vi "Zero-Pole (DBL).vi"(2 "initialize":bool, 3 "dt":dbl=1e-09 min=1e-09 format="%.6f", 4 "gain-zeros-poles":T1 {"Poles" format="%.2f"; "Zeros" format="%.2f"; "gain" format="%.2f"}, 5 "input point":dbl format="%.2f") -> (1 "output point":dbl format="%.2f")   [LabVIEW 2017, in "NI_AdvCtrl_continuous linear.lvlib"]
doc: "LabVIEW no longer supports this VI. You can obtain similar functionality by installing the LabVIEW Simulation Module.\n\nCalculates the new output point, where the transfer function and the input point are given. The transfer function is described in gain-zeros-poles notation."
uses:
  <vilib>/addons/control/advanced/NI_AdvCtrl_continuous linear.lvlib
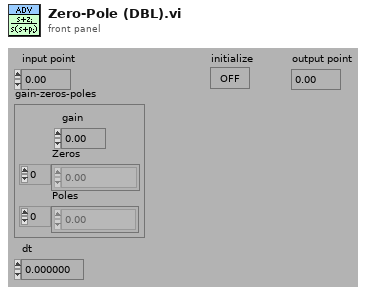
[diagram p1: front panel]
types:
  T1 = cluster{"gain":dbl, "Zeros":cdb[], "Poles":cdb[]}
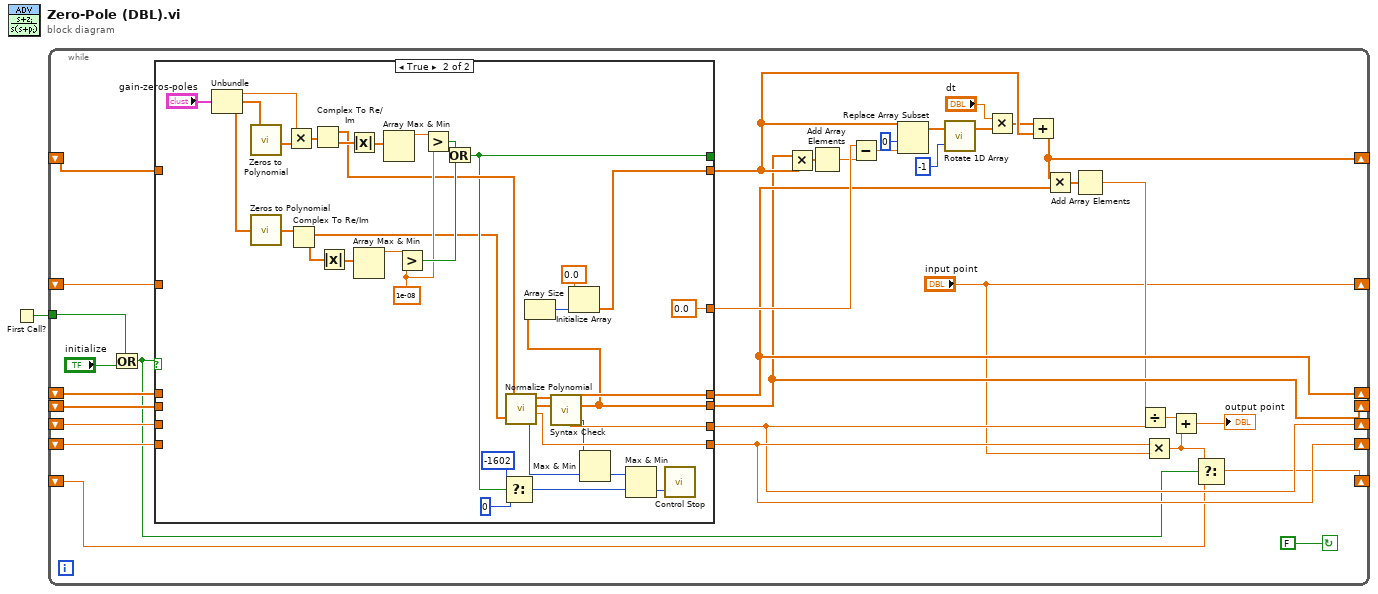
[diagram p0: block diagram]
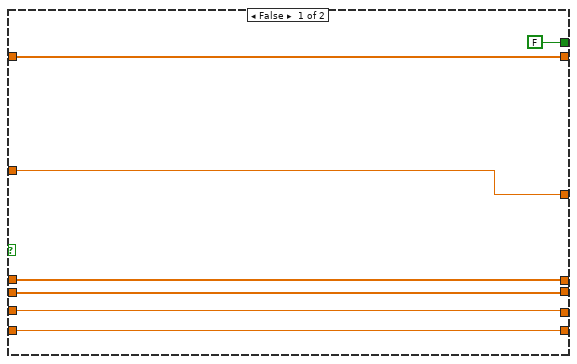
[diagram p2: hidden frame]
diagram:
  n1 = First Call?() -> (First Call?: T/F=w1:bool)
  n2 = while {
    shift-left: _ -> [w24]
    shift-right: ["input point"] -> _
    shift-left: _ -> [w26]
    shift-right: [w22] -> _
    tunnel: w1 -> [w27]
    shift-left: _ -> [w9]
    shift-right: [w6] -> _
    shift-left: _ -> [w32]
    shift-right: [w31] -> _
    shift-left: _ -> [w33]
    shift-right: [w30] -> _
    shift-left: _ -> [w34]
    shift-right: [w20] -> _
    shift-left: _ -> [w35]
    shift-right: [w21] -> _
    stop <- FALSE continue-if-true
    n3 = Or(x=w27, y="initialize") -> (x .or. y?=w8:bool)
    n4 = case shown="True" w8 {
      tunnel: [w39 w78] -> w31
      tunnel: [w40 w75] -> w30
      tunnel: [w42 w74] -> w21
      tunnel: [w41 w43] -> w20
      tunnel: w35 -> [w42 _]
      tunnel: w34 -> [w41 _]
      tunnel: w33 -> [w40 _]
      tunnel: w32 -> [w39 _]
      tunnel: [w38 w46] -> w23
      tunnel: w26 -> [w38 _]
      tunnel: [w37 0.0 ("input point")] -> w25
      tunnel: w24 -> [w37 _]
      tunnel: [FALSE w51] -> _
      frame False {
      }
      frame True {
        w66 = 1e-08
        n5 = Unbundle("gain-zeros-poles") -> ("gain"=w55:dbl, "Zeros"=w58:cdb[], "Poles"=w57:cdb[])
        n6 = call <vilib>:"Zeros to Polynomial.vi"("Zeros"=w58) -> ("Polynomial"=w56:cdb[])
        n7 = call <vilib>:"Zeros to Polynomial.vi"("Zeros"=w57) -> ("Polynomial"=w62:cdb[])
        n8 = Multiply(x=w55, y=w56) -> (x*y=w61:cdb[])
        n9 = Complex To Re/Im(x + iy=w62) -> (x=w44:dbl[], y=w64:dbl[])
        n10 = Complex To Re/Im(x + iy=w61) -> (x=w60:dbl[], y=w70:dbl[])
        n11 = Absolute Value(x=w64) -> (abs(x)=w63:dbl[])
        n12 = Absolute Value(x=w70) -> (abs(x)=w69:dbl[])
        n13 = Array Max & Min(array=w63) -> (max value=w65:dbl)  [unwired: 3 out]
        n14 = Array Max & Min(array=w69) -> (max value=w71:dbl)  [unwired: 3 out]
        n15 = Greater?(x=w65, y=w66) -> (0:w67:bool)
        n16 = Greater?(x=w71, y=w66) -> (0:w68:bool)
        n17 = Or(x=w68, y=w67) -> (x .or. y?=w51:bool)
        n18 = Select(t=-1602, s=w51, f=0) -> (s? t:f=w48:i32)
        n19 = call <vilib>:"Normalize Polynomial.vi"("Numerator"=w60, "Denominator"=w44) -> ("Numerator new"=w76:dbl[], "Denominator new"=w77:dbl[], "additive constant"=w78:dbl, "error"=w53:i32)
        n20 = call <vilib>:"Syntax Check.vi"("Denominator"=w77, "Numerator"=w76) -> ("error"=w54:i32, "gain"=w75:dbl, "Denominator new"=w43:dbl[], "Numerator new"=w74:dbl[])  [unwired: 1 out]
        n21 = Array Size(array=w43) -> (size(s)=w72:i32)
        n22 = Initialize Array(0.0, w72) -> (w46:dbl[])
        n23 = Max & Min(x=w54, y=w53) -> (min(x,y)=w52:i32)  [unwired: 1 out]
        n24 = Max & Min(x=w52, y=w48) -> (min(x,y)=w47:i32)  [unwired: 1 out]
        n25 = call <vilib>:"Control Stop.vi"("error"=w47) -> ()  [unwired: 2 out]
      }
    }
    n26 = Multiply(x=w20, y=w23) -> (x*y=w17:dbl[])
    n27 = Add Array Elements(numeric array=w17) -> (sum=w16:dbl)
    n28 = Subtract(x=w25, y=w16) -> (x-y=w19:dbl)
    n29 = Replace Array Subset(array=w23, new element=w19, index=0 ("Index")) -> (w5:dbl[])
    n30 = call <vilib>:"Rotate 1D Array.vi"("n"=-1, "array"=w5) -> ("array (last n elements first)"=w3:dbl[])  [unwired: 1 out]
    n31 = Multiply(x="dt", y=w3) -> (x*y=w15:dbl[])
    n32 = Add(x=w15, y=w23) -> (x+y=w22:dbl[])
    n33 = Multiply(x=w22, y=w21) -> (x*y=w14:dbl[])
    n34 = Add Array Elements(numeric array=w14) -> (sum=w13:dbl)
    n35 = Divide(x=w13, y=w30) -> (x/y=w11:dbl)
    n36 = Multiply(x=w31, y="input point") -> (x*y=w7:dbl)
    n37 = Add(x=w11, y=w7) -> (x+y=→"output point":dbl)
    n38 = Select(t=w7, s=w8, f=w9) -> (s? t:f=w6:dbl)
  }
